vi "Aprox Equal Zero.vi"(9 "epsilion":dbl=0.05, 10 "x":dbl) -> (2 "Boolean":bool)   [LabVIEW 2025]
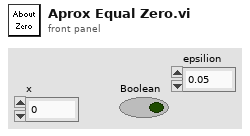
[diagram p1: front panel]
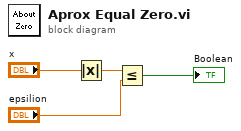
[diagram p0: block diagram]
diagram:
  n1 = Absolute Value(x="x") -> (abs(x)=w3:dbl)
  n2 = Less Or Equal?(x=w3, y="epsilion") -> (x <= y?=→"Boolean":bool)
